vi "JPL Button Cycler.vi"(3 "# Switch Outputs":dbl, 5 "Switch Input":bool) -> (1 "Switch Output":T1)   [LabVIEW 2014]
uses:
  <vilib>/functionblocks/Edge Detection/One Shot Rising with Input/One Shot Rising with Input.vi
  <vilib>/functionblocks/FB Core/FB Core.xnode
  <vilib>/functionblocks/NI_FunctionBlock Libraries.lvlib
panel:
  out "Index":dbl
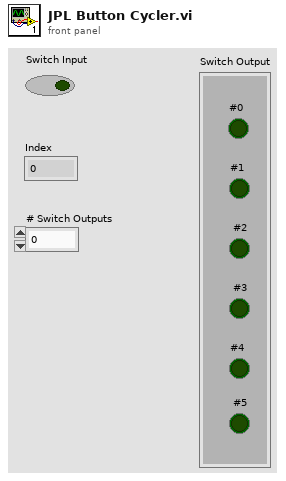
[diagram p1: front panel]
types:
  T1 = cluster{"#0":bool, "#1":bool, " #2":bool, " #3":bool, "#4":bool, " #5":bool}
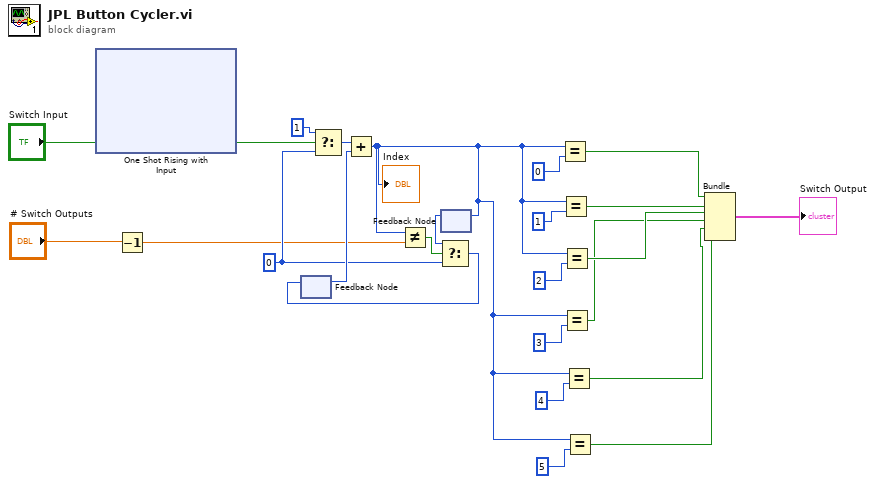
[diagram p0: block diagram]
diagram:
  w19 = 0
  n1 = xnode "One Shot Rising with Input"("input"="Switch Input") -> ("output"=w18:bool)  [unwired: 1 in, 1 out]
  n2 = Decrement(x="# Switch Outputs") -> (x-1=w10:dbl)
  n3 = feedback #1() -> (w21:i32)  [unwired: 1 in]
  n4 = Select(t=1, s=w18, f=w19) -> (s? t:f=w24:i32)
  n5 = Add(x=w24, y=w21) -> (x+y=w4:i32)
  "Index" <- w4
  n6 = Not Equal?(x=w4, y=w10) -> (x != y?=w23:bool)
  n7 = feedback #2() -> (w20:i32)  [unwired: 1 in]
  n8 = Select(t=w20, s=w23, f=w19) -> (s? t:f=w22:i32)
  n9 = feedback-in #1(w22) -> ()
  n10 = feedback-in #2(w4) -> ()
  n11 = Equal?(x=w4, y=0) -> (x = y?=w14:bool)
  n12 = Equal?(x=w4, y=1) -> (x = y?=w13:bool)
  n13 = Equal?(x=w4, y=2) -> (x = y?=w12:bool)
  n14 = Equal?(x=w4, y=3) -> (x = y?=w7:bool)
  n15 = Equal?(x=w4, y=4) -> (x = y?=w3:bool)
  n16 = Equal?(x=w4, y=5) -> (x = y?=w2:bool)
  n17 = Bundle(w14, w13, w12, w7, w3, w2) -> (→"Switch Output":cluster{bool, bool, bool, bool, bool, bool})  [unwired: 1 in]
